vi "PI_Image_Scanner_Prepare_Dlg.vi"(0 "System no.":i32, 5 "Image Measurent Parameters":T1, 7 "Line Scan":bool, 9 "LineScan Cycles":u16, 11 "error in":errorcluster, 12 "Learning loop":bool=TRUE) -> (4 "System no. (dup)":i32, 8 "Measurement time [s]":dbl, 15 "error out":errorcluster)   [LabVIEW 2011]
panel:
  out "Programming scanner":u8(slide) caption="Preparing Scanner" scale=0.0..100.0
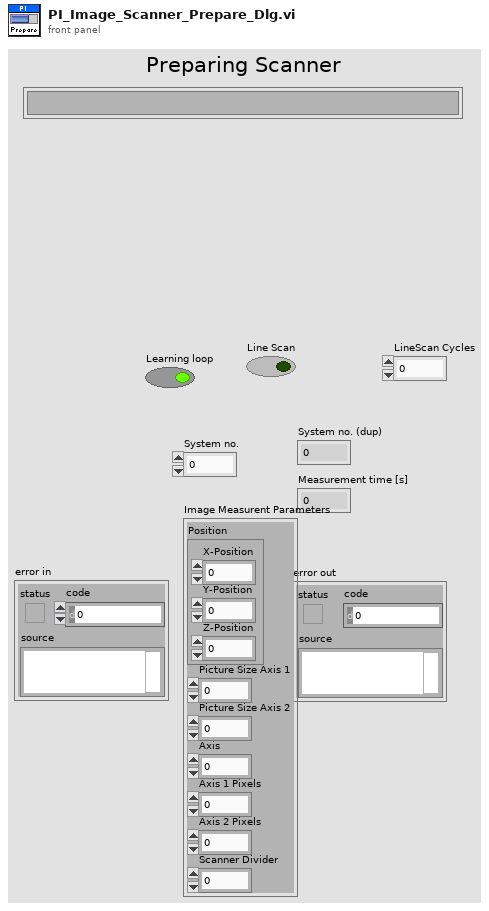
[diagram p1: front panel]
types:
  T1 = cluster{"Position":cluster{"X-Position":dbl, "Y-Position":dbl, "Z-Position":dbl}, "Picture Size Axis 1":dbl, "Picture Size Axis 2":dbl, "Axis":i32, "Axis 1 Pixels":u16, "Axis 2 Pixels":u16, "Scanner Divider":i32}
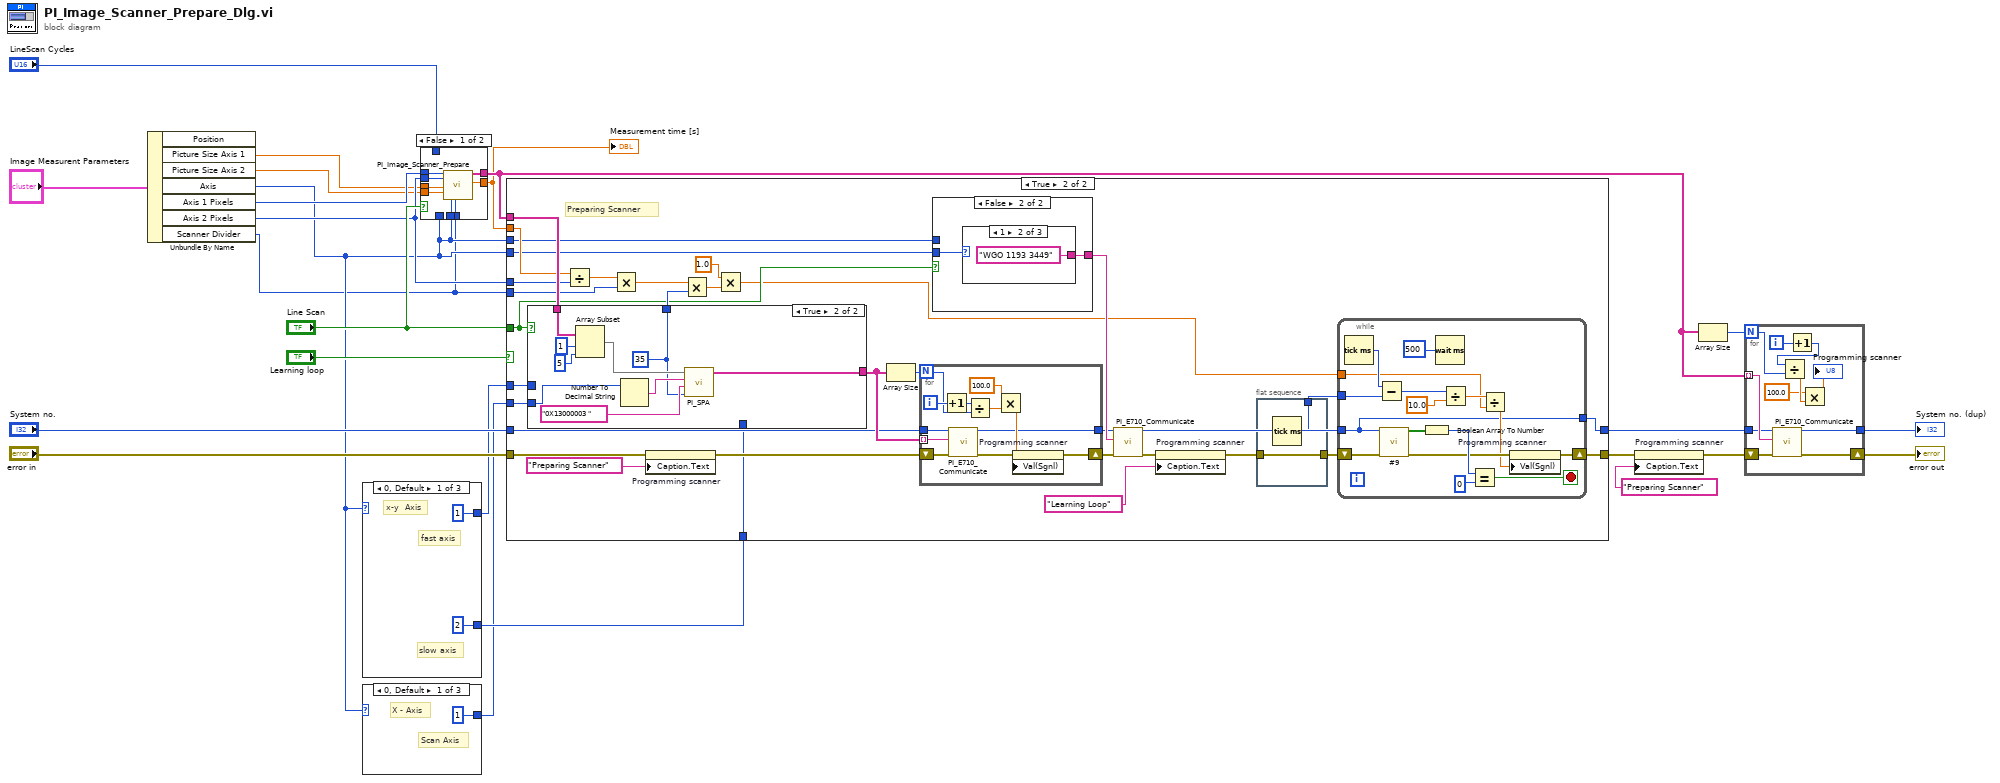
[diagram p0: block diagram]
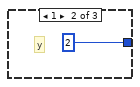
[diagram p2: hidden frame]
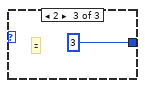
[diagram p3: hidden frame]
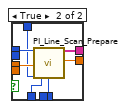
[diagram p4: hidden frame]
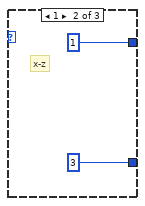
[diagram p5: hidden frame]
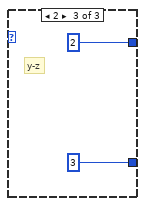
[diagram p6: hidden frame]
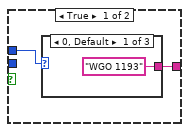
[diagram p8: hidden frame]
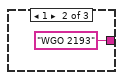
[diagram p9: hidden frame]
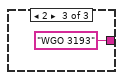
[diagram p10: hidden frame]
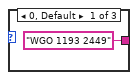
[diagram p11: hidden frame]
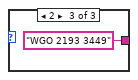
[diagram p12: hidden frame]
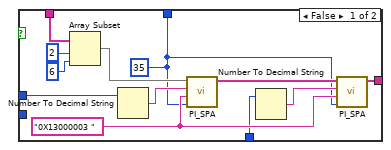
[diagram p13: hidden frame]
diagram:
  n1 = Unbundle By Name("Image Measurent Parameters") -> ("Picture Size Axis 1"=w4:dbl, "Picture Size Axis 2"=w3:dbl, "Axis"=w2:i32, "Axis 1 Pixels"=w6:u16, "Axis 2 Pixels"=w5:u16, "Scanner Divider"=w1:i32)  [unwired: 1 out]
  n2 = case shown="0, Default" w2 {
    tunnel: [1 1 2] -> w12
    tunnel: [2 3 3] -> w11
    frame 0, Default {
      # "x-y  Axis"
      # "slow axis"
      # "fast axis"
    }
    frame 1 {
      # "x-z"
    }
    frame 2 {
      # "y-z"
    }
  }
  n3 = case shown="0, Default" w2 {
    tunnel: [1 2 3] -> w8
    frame 0, Default {
      # "X - Axis"
      # "Scan Axis"
    }
    frame 1 {
      # "y"
    }
    frame 2 {
      # "z"
    }
  }
  n4 = case shown="False" "Line Scan" {
    tunnel: w1 -> [w41 w43]
    tunnel: w4 -> [w40 w45]
    tunnel: w3 -> [w39 _]
    tunnel: w6 -> [w38 w46]
    tunnel: [w37 w48] -> w19
    tunnel: [w36 w47] -> w18
    tunnel: w5 -> [w35 _]
    tunnel: w2 -> [w34 _]
    tunnel: w2 -> [_ w44]
    tunnel: "LineScan Cycles" -> [_ w42]
    frame False {
      n5 = call "PI_Image_Scanner_Prepare.vi"("x-Pixel"=w38, "y-Pixel"=w35, "Picture size x"=w40, "Picture size y"=w39, "Axis"=w34, "Scanner Divider"=w41) -> ("Commandset out"=w37:string[], "Measurement time / [s]"=w36:dbl)  [unwired: 12 in]
    }
    frame True {
      n6 = call "PI_Line_Scan_Prepare.vi"("Pixel"=w46, "Line Length"=w45, "Wave Cycles"=w42, "Axis"=w44, "Scanner Divider"=w43) -> ("Commandset out"=w48:string[], "Measurement time / [s]"=w47:dbl)  [unwired: 13 in]
    }
  }
  "Measurement time [s]" <- w18
  n7 = case shown="True" "Learning loop" {
    tunnel: w19 -> [_ w82]
    tunnel: w18 -> [_ w76]
    tunnel: w2 -> [_ w70]
    tunnel: w5 -> [_ w69]
    tunnel: "System no." -> [w49 w68]
    tunnel: "error in" -> [w50 w67]
    tunnel: [w50 w63] -> w15
    tunnel: [w49 w62] -> w13
    tunnel: w12 -> [_ w61]
    tunnel: w11 -> [_ w60]
    tunnel: w1 -> [_ w59]
    tunnel: "Line Scan" -> [_ w55]
    tunnel: w8 -> [_ w56]
    tunnel: w2 -> [_ w54]
    frame False {
    }
    frame True {
      # "Preparing Scanner"
      n8 = case shown="True" w55 {
        tunnel: w82 -> [w105 w114]
        tunnel: [w97 w108] -> w80
        tunnel: [w96 w109] -> w77
        tunnel: w61 -> [w95 _]
        tunnel: w60 -> [w94 _]
        tunnel: w56 -> [_ w107]
        frame False {
          w96 = u16 35 ("Value")
          w98 = "0X13000003 " ("string")
          n9 = Array Subset(array=w105, index=2 ("Index"), length=6 ("Länge")) -> (w102:string[])
          n10 = Number To Decimal String(number=w95) -> (decimal integer string=w100:string)  [unwired: 1 out]
          n11 = call "PI_SPA.vi"("Value"=w96, "Register"=w98, "Axis"=w100, "Commandset in"=w102) -> ("Commandset out"=w101:string[])  [unwired: 7 out]
          n12 = Number To Decimal String(number=w94) -> (decimal integer string=w99:string)  [unwired: 1 out]
          n13 = call "PI_SPA.vi"("Value"=w96, "Register"=w98, "Axis"=w99, "Commandset in"=w101) -> ("Commandset out"=w97:string[])  [unwired: 7 out]
        }
        frame True {
          w109 = u16 35 ("Value")
          n14 = Array Subset(array=w114, index=1, length=5 ("Länge")) -> (w112:string[])
          n15 = Number To Decimal String(number=w107) -> (decimal integer string=w111:string)  [unwired: 1 out]
          n16 = call "PI_SPA.vi"("Value"=w109, "Register"="0X13000003 " ("string"), "Axis"=w111, "Commandset in"=w112) -> ("Commandset out"=w108:string[])  [unwired: 7 out]
        }
      }
      n17 = Divide(x=w76, y=w69) -> (x/y=w58:dbl)
      n18 = Multiply(x=w58, y=w59) -> (x*y=w57:dbl)
      n19 = property on="Programming scanner" class="Slide (strict)"(error in=w67, "Caption.Text"="Preparing Scanner" ("Beschriftung.Text")) -> (error out=w74:errorcluster)  [unwired: 1 in, 1 out]
      n20 = Multiply(x=w57, y=w77) -> (x*y=w53:dbl)
      n21 = Multiply(x=1.0, y=w53) -> (x*y=w52:dbl)
      n22 = Array Size(array=w80) -> (size(s)=w79:i32)
      n23 = for {
        N: w79 -> [w141]
        tunnel: w80 -> [w144] mode=indexing
        tunnel: [w137] -> w78
        shift-right: [w134] -> w83
        shift-left: w74 -> [w136]
        tunnel: w68 -> [w133]
        i -> [w143]
        n24 = Increment(x=w143) -> (x+1=w142:i32)
        n25 = call "PI_E710_Communicate.vi"("System no."=w133, "String to send"=w144, "error in"=w136) -> ("System no. (dup)"=w137:i32, "error out"=w135:errorcluster)  [unwired: 14 in, 1 out]
        n26 = Divide(x=w142, y=w141) -> (x/y=w140:dbl)
        n27 = Multiply(x=100.0, y=w140) -> (x*y=w138:dbl)
        n28 = property on="Programming scanner" class="Slide (strict)"(error in=w135, "Val(Sgnl)"=w138) -> (error out=w134:errorcluster)  [unwired: 1 in, 1 out]
      }
      n29 = case shown="False" w55 {
        tunnel: [w85 w90] -> w81
        tunnel: w70 -> [_ w89]
        tunnel: w54 -> [w84 _]
        frame True {
          n30 = case shown="0, Default" w84 {
            tunnel: ["WGO 1193" ("String to send") "WGO 2193" ("String to send") "WGO 3193" ("String to send")] -> w85
            frame 0, Default {
            }
            frame 1 {
            }
            frame 2 {
            }
          }
        }
        frame False {
          n31 = case shown="1" w89 {
            tunnel: ["WGO 1193 2449" ("String to send") "WGO 1193 3449" ("String to send") "WGO 2193 3449" ("String to send")] -> w90
            frame 0, Default {
            }
            frame 1 {
            }
            frame 2 {
            }
          }
        }
      }
      n32 = call "PI_E710_Communicate.vi"("System no."=w78, "String to send"=w81, "error in"=w83) -> ("System no. (dup)"=w71:i32, "error out"=w73:errorcluster)  [unwired: 14 in, 1 out]
      n33 = property on="Programming scanner" class="Slide (strict)"(error in=w73, "Caption.Text"="Learning Loop" ("Beschriftung.Text")) -> (error out=w66:errorcluster)  [unwired: 1 in, 1 out]
      n34 = flat-sequence {
        tunnel: w66 -> [w116]
        tunnel: [w116] -> w65
        tunnel: [w115] -> w64
        frame #0 {
          n35 = Tick Count (ms)() -> (millisecond timer value=w115:u32)
        }
      }
      n36 = while {
        tunnel: w71 -> [w117]
        tunnel: w52 -> [w126]
        tunnel: w64 -> [w127]
        shift-right: [w118] -> w63
        shift-left: w65 -> [w125]
        tunnel: [w117] -> w62
        stop <- w121 stop-if-true
        n37 = Tick Count (ms)() -> (millisecond timer value=w131:u32)
        n38 = Subtract(x=w131, y=w127) -> (x-y=w130:u32)
        n39 = call <userlib>:"#9.vi"("System no."=w117, "error in"=w125) -> ("WG running?"=w124:bool[], "error out"=w120:errorcluster)  [unwired: 16 in]
        n40 = Boolean Array To Number(Boolean array=w124) -> (number=w123:u32)
        n41 = Wait (ms)(milliseconds to wait=u32 500 ("Zu wartende ms")) -> ()  [unwired: 1 out]
        n42 = Divide(x=w130, y=10.0) -> (x/y=w128:dbl)
        n43 = Equal?(x=w123, y=u32 0) -> (x = y?=w121:bool)
        n44 = Divide(x=w128, y=w126) -> (x/y=w119:dbl)
        n45 = property on="Programming scanner" class="Slide (strict)"(error in=w120, "Val(Sgnl)"=w119) -> (error out=w118:errorcluster)  [unwired: 1 in, 1 out]
      }
    }
  }
  n46 = property on="Programming scanner" class="Slide (strict)"(error in=w15, "Caption.Text"="Preparing Scanner" ("Label.Text")) -> (error out=w21:errorcluster)  [unwired: 1 in, 1 out]
  n47 = Array Size(array=w19) -> (size(s)=w22:i32)
  n48 = for {
    N: w22 -> [w153]
    tunnel: w19 -> [w149] mode=indexing
    shift-right: [w147] -> w24
    shift-left: w21 -> [w148]
    tunnel: w13 -> [w146]
    tunnel: [w145] -> w23
    i -> [w155]
    n49 = call "PI_E710_Communicate.vi"("System no."=w146, "String to send"=w149, "error in"=w148) -> ("System no. (dup)"=w145:i32, "error out"=w147:errorcluster)  [unwired: 14 in, 1 out]
    n50 = Increment(x=w155) -> (x+1=w154:i32)
    n51 = Divide(x=w154, y=w153) -> (x/y=w152:dbl)
    n52 = Multiply(x=100.0, y=w152) -> (x*y=→"Programming scanner":dbl)
  }
  "error out" <- w24
  "System no. (dup)" <- w23
